vi "Init.vi"(8 "error in (no error)":errorcluster, 10 "Channel":i16, 11 "TrialBasedExperiment in":refnum<class "ClassDiscrimination.lvclass">) -> (0 "error out":errorcluster, 3 "TrialBasedExperiment out":refnum<class "ClassDiscrimination.lvclass">)   [LabVIEW 2010, in "ClassDiscrimination.lvclass"]
uses:
  ClassDiscrimination.lvclass
  MatlabExperiment/MatlabExperiment.lvclass
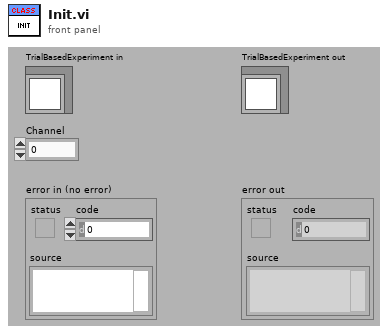
[diagram p1: front panel]
types:
  T1 = cluster{"Intertrial":dbl, "AcquireFixation":dbl, "HoldFixation":dbl, "DelayPeriod":dbl, "ResponsePeriod":dbl}
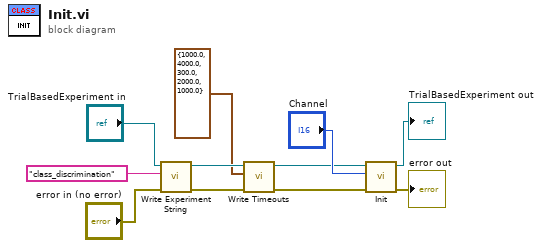
[diagram p0: block diagram]
diagram:
  n1 = call-dynamic "Write Experiment String.vi"("error in (no error)"="error in (no error)", "Experiment String"="class_discrimination", "TrialBasedExperiment in"="TrialBasedExperiment in") -> ("error out"=w4:errorcluster, "TrialBasedExperiment out"=w5:refnum<class "ClassDiscrimination.lvclass">)  [unwired: 7 in]
  n2 = call-dynamic "Write Timeouts.vi"("error in (no error)"=w4, "Timeouts"=T1 {"Intertrial"=1000.0, "AcquireFixation"=4000.0, "HoldFixation"=300.0, "DelayPeriod"=2000.0, "ResponsePeriod"=1000.0}, "TrialBasedExperiment in"=w5) -> ("error out"=w3:errorcluster, "TrialBasedExperiment out"=w2:refnum<class "ClassDiscrimination.lvclass">)  [unwired: 7 in]
  n3 = call-parent "Init.vi"("error in (no error)"=w3, "Channel"="Channel", "TrialBasedExperiment in"=w2) -> ("error out"=→"error out":errorcluster, "TrialBasedExperiment out"=→"TrialBasedExperiment out":refnum<class "ClassDiscrimination.lvclass">)  [unwired: 7 in]
